vi "Calibration Parameter Add_Modify - UI.vi"(8 "Error In":errorcluster, 9 "Parameter List":string[](array[string]), 10 "Add??":bool, 11 "Parameter Details In":T1) -> (0 "Error Out":errorcluster, 2 "Processed":bool, 3 "Parameter Details Out":T1)   [LabVIEW 2010]
uses:
  Calibration dates.ctl
panel:
  out "Welcome String":string
  in  "Corrections":dbl format="%#.2f"
  in  "Parameter Type":string
  in  "Last Calibrated Date":timestamp=timestamp(3296822614.6226506 s since 1904-01-01) format="%<%x>T"
  in  "Calibration Due Date":timestamp=timestamp(3296822614.6226506 s since 1904-01-01) format="%<%x>T"
  in  "Exit":bool
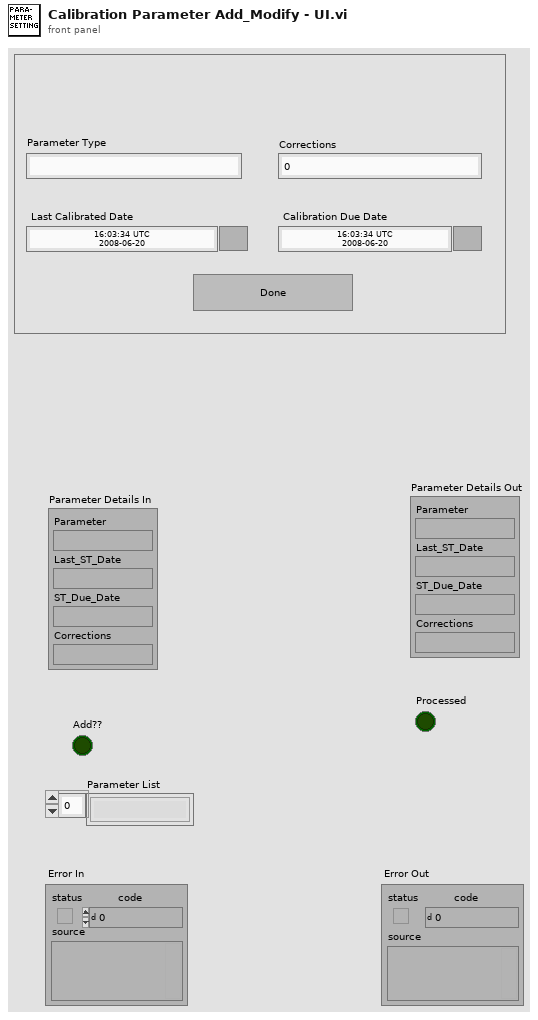
[diagram p1: front panel]
types:
  T1 = typedef "Calibration dates.ctl" = cluster{"Parameter":string, "Last_ST_Date":string, "ST_Due_Date":string, "Corrections":string}
  T2 = typedef "LVDateTimeRec.ctl" = cluster{"fractional second":dbl, "second":i32, "minute":i32, "hour":i32, "day of month":i32, "month":i32, "year":i32, "day of week":i32, "day of year":i32, "DST":i32}
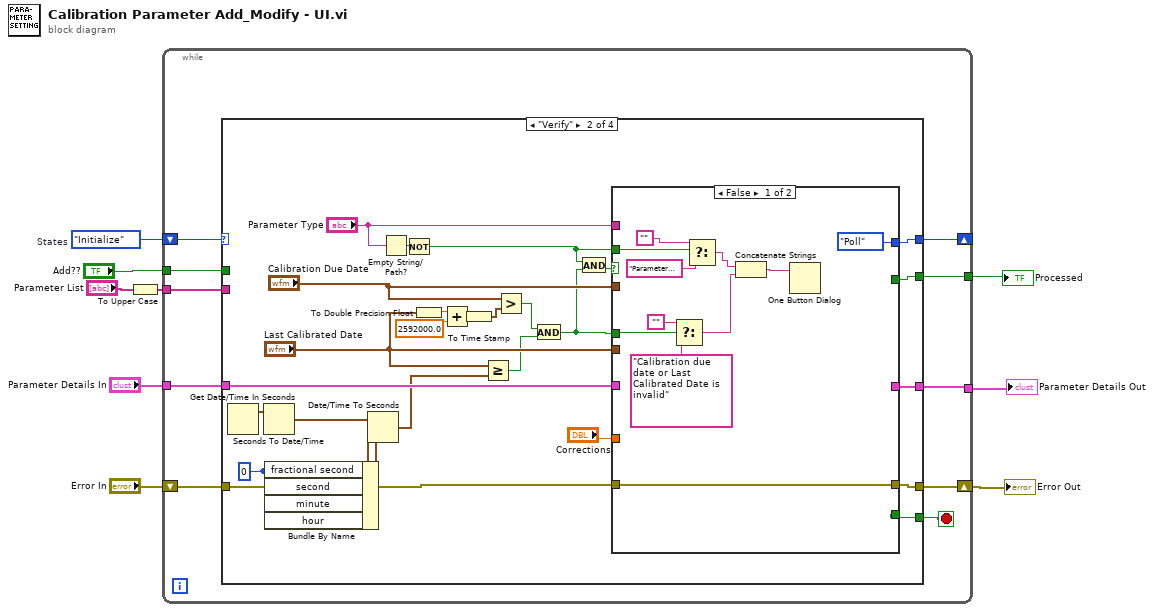
[diagram p0: block diagram]
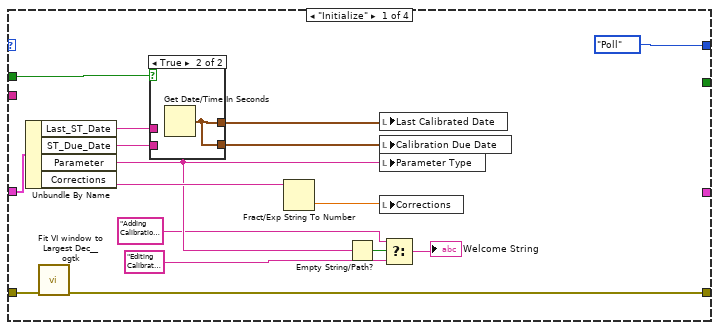
[diagram p2: hidden frame]
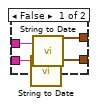
[diagram p3: hidden frame]
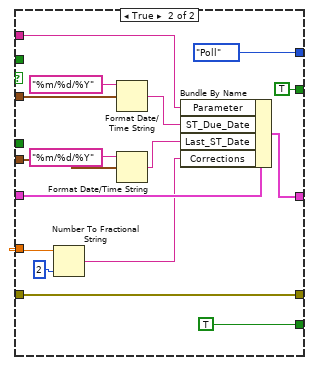
[diagram p4: hidden frame]
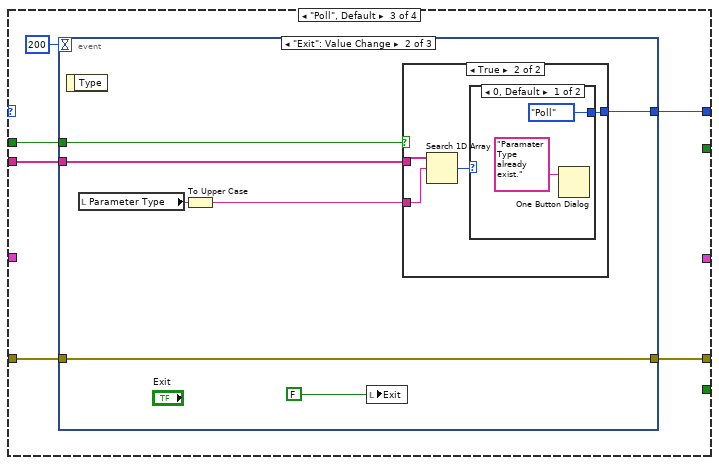
[diagram p5: hidden frame]
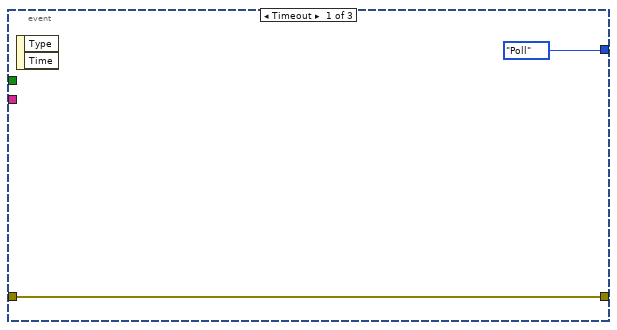
[diagram p6: hidden frame]
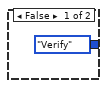
[diagram p7: hidden frame]
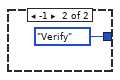
[diagram p8: hidden frame]
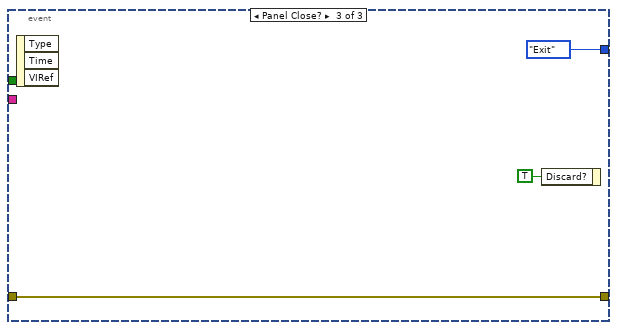
[diagram p9: hidden frame]
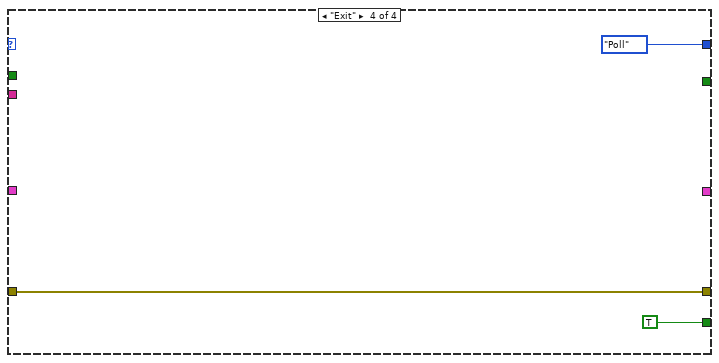
[diagram p10: hidden frame]
diagram:
  w9 = enum16{"Poll", "Initialize", "Verify", "Exit"}."Initialize"  # States
  n1 = To Upper Case(1:"Parameter List") -> (0:w1:string[])
  n2 = while {
    shift-right: [w18] -> _
    shift-left: w9 -> [w19]
    shift-right: [w15] -> w7
    shift-left: "Error In" -> [w16]
    tunnel: "Parameter Details In" -> [w14]
    tunnel: [w13] -> w5
    tunnel: [w12] -> w4
    tunnel: w1 -> [w11]
    tunnel: "Add??" -> [w10]
    stop <- w17 stop-if-true
    n3 = case shown="\"Verify\"" w19 {
      tunnel: [enum16{"Poll", "Initialize", "Verify", "Exit"}."Poll" ("States") w66 w98 enum16{"Poll", "Initialize", "Verify", "Exit"}."Poll" ("States")] -> w18
      tunnel: [_ w61 _ TRUE] -> w17
      tunnel: w16 -> [w35 w64 w97 w121]
      tunnel: [w34 w63 w96 w121] -> w15
      tunnel: w14 -> [w33 w57 _ _]
      tunnel: [_ w56 _ _] -> w13
      tunnel: [_ w55 _ _] -> w12
      tunnel: w11 -> [_ _ w95 _]
      tunnel: w10 -> [w20 _ w94 _]
      frame "Initialize" {
        n4 = Unbundle By Name(w33) -> ("Last_ST_Date"=w22:string, "ST_Due_Date"=w21:string, "Parameter"=w28:string, "Corrections"=w30:string)
        n5 = call <userlib>:"Fit VI window to Largest Dec__ogtk.vi"("error in (no error)"=w35) -> ("error out"=w34:errorcluster)  [unwired: 5 in, 1 out]
        n6 = case shown="True" w20 {
          tunnel: [w39 w40] -> w32
          tunnel: [w38 w40] -> w31
          tunnel: w22 -> [w37 _]
          tunnel: w21 -> [w36 _]
          frame False {
            n7 = call "String to Date.vi"("Cal Due Date"=w36) -> ("time stamp"=w38:timestamp)  [unwired: 10 in]
            n8 = call "String to Date.vi"("Cal Due Date"=w37) -> ("time stamp"=w39:timestamp)  [unwired: 10 in]
          }
          frame True {
            n9 = Get Date/Time In Seconds() -> (seconds since 1Jan1904=w40:timestamp)
          }
        }
        n10 = Fract/Exp String To Number(string=w30) -> (number=w29:dbl)  [unwired: 3 in, 1 out]
        n11 = Empty String/Path?(string/path=w28) -> (empty?=w27:bool)
        n12 = local write "Last Calibrated Date"(w32) -> ()
        n13 = local write "Calibration Due Date"(w31) -> ()
        n14 = local write "Parameter Type"(w28) -> ()
        n15 = local write "Corrections"(w29) -> ()
        n16 = Select(t="Adding Calibration Parameter" ("Parameter"), s=w27, f="Editing Calibration Parameter" ("Parameter")) -> (s? t:f=→"Welcome String":string)
      }
      frame "Verify" {
        w41 = 0 ("hour")
        n17 = Get Date/Time In Seconds() -> (seconds since 1Jan1904=w43:timestamp)
        n18 = Seconds To Date/Time(time stamp (now)=w43) -> (date time rec=w45:T2)  [unwired: 1 in]
        n19 = Bundle By Name(cluster=w45, "fractional second"=w41, "second"=w41, "minute"=w41, "hour"=w41) -> (w44:T2)
        n20 = Date/Time To Seconds(2:w44) -> (0:w42:timestamp)  [unwired: 1 in]
        n21 = Empty String/Path?(string/path="Parameter Type") -> (empty?=w65:bool)
        n22 = Not(x=w65) -> (.not. x?=w54:bool)
        n23 = To Double Precision Float(number="Last Calibrated Date") -> (double precision float=w51:dbl)
        n24 = Add(x=w51, y=2592000.0) -> (x+y=w52:dbl)
        n25 = To Time Stamp(1:w52) -> (0:w50:timestamp)
        n26 = Greater Or Equal?(x="Last Calibrated Date", y=w42) -> (x >= y?=w47:bool)
        n27 = Greater?(x="Calibration Due Date", y=w50) -> (0:w48:bool)
        n28 = And(x=w48, y=w47) -> (x .and. y?=w46:bool)
        n29 = And(x=w54, y=w46) -> (x .and. y?=w62:bool)
        n30 = case shown="False" w62 {
          tunnel: [enum16{"Poll", "Initialize", "Verify", "Exit"}."Poll" ("States") enum16{"Poll", "Initialize", "Verify", "Exit"}."Poll" ("States")] -> w66
          tunnel: [w77 w93] -> w63
          tunnel: w64 -> [w77 w93]
          tunnel: [_ TRUE] -> w61
          tunnel: "Corrections" -> [_ w86]
          tunnel: "Last Calibrated Date" -> [_ w89]
          tunnel: "Calibration Due Date" -> [_ w87]
          tunnel: "Parameter Type" -> [_ w79]
          tunnel: w57 -> [_ w84]
          tunnel: [_ w81] -> w56
          tunnel: [_ TRUE] -> w55
          tunnel: w46 -> [w73 _]
          tunnel: w54 -> [w75 _]
          frame False {
            n31 = Select(t="", s=w73, f="Calibration due date or Last Calibrated Date is invalid" ("Parameter Type")) -> (s? t:f=w70:string)
            n32 = Select(t="", s=w75, f="Parameter Type is Empty\\null.\n" ("Parameter Type")) -> (s? t:f=w69:string)
            n33 = Concatenate Strings(w69, w70) -> (w68:string)
            n34 = One Button Dialog(message=w68) -> ()  [unwired: 1 in, 1 out]
          }
          frame True {
            n35 = Number To Fractional String(number=w86, precision (6)=i16 2) -> (F-format string=w83:string)  [unwired: 2 in]
            n36 = Format Date/Time String(time format string (%c)="%m/%d/%Y", seconds (now)=w87) -> (date/time string=w80:string)  [unwired: 1 in]
            n37 = Format Date/Time String(time format string (%c)="%m/%d/%Y", seconds (now)=w89) -> (date/time string=w82:string)  [unwired: 1 in]
            n38 = Bundle By Name(cluster=w84, "Parameter"=w79, "ST_Due_Date"=w80, "Last_ST_Date"=w82, "Corrections"=w83) -> (w81:T1)
          }
        }
      }
      frame "Poll", Default {
        n39 = event shown="[1] \"Exit\": Value Change" {
          selector: _ -> [_ _ _]
          dyn-events: _ -> [_ _ _]
          timeout: 200 -> [_ _ _]
          tunnel: [enum16{"Poll", "Initialize", "Verify", "Exit"}."Poll" ("States") w107 enum16{"Poll", "Initialize", "Verify", "Exit"}."Exit" ("States")] -> w98
          tunnel: w97 -> [w101 w108 w119]
          tunnel: [w101 w108 w119] -> w96
          tunnel: w95 -> [_ w102 _]
          tunnel: w94 -> [_ w104 _]
          event Timeout {
            n40 = event-data() -> ()  [unwired: 1 in, 2 out]
          }
          event "Exit": Value Change {
            n41 = event-data() -> ()  [unwired: 1 in, 1 out]
            n42 = local read "Parameter Type"() -> (w105:string)
            n43 = To Upper Case(1:w105) -> (0:w103:string)
            n44 = local write "Exit"(FALSE ("Exit")) -> ()
            n45 = case shown="True" w104 {
              tunnel: [enum16{"Poll", "Initialize", "Verify", "Exit"}."Verify" ("States") w110] -> w107
              tunnel: w103 -> [_ w112]
              tunnel: w102 -> [_ w113]
              frame False {
              }
              frame True {
                n46 = Search 1D Array(1D array=w113, element=w112) -> (index of element=w111:i32)  [unwired: 1 in]
                n47 = case shown="0, Default" w111 {
                  tunnel: [enum16{"Poll", "Initialize", "Verify", "Exit"}."Poll" ("States") enum16{"Poll", "Initialize", "Verify", "Exit"}."Verify" ("States")] -> w110
                  frame 0, Default {
                    n48 = One Button Dialog(message="Paramater Type already exist.") -> ()  [unwired: 1 in, 1 out]
                  }
                  frame -1 {
                  }
                }
              }
            }
          }
          event Panel Close? {
            n49 = event-data() -> ()  [unwired: 1 in, 3 out]
            n50 = event-data("Discard?"=TRUE) -> ()  [unwired: 1 in, 1 out]
          }
        }
      }
      frame "Exit" {
      }
    }
  }
  "Error Out" <- w7
  "Parameter Details Out" <- w5
  "Processed" <- w4
